vi "Startup Serial Packet Read.vi"(0 "VISA resource In":refnum<visa-resource-name>, 7 "End Character":string, 11 "error in":errorcluster) -> (4 "VISA resource Out":refnum<visa-resource-name>, 8 "Data Out":string, 15 "error out":errorcluster)   [LabVIEW 2014]
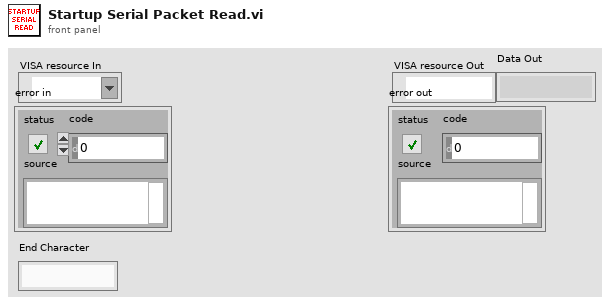
[diagram p1: front panel]
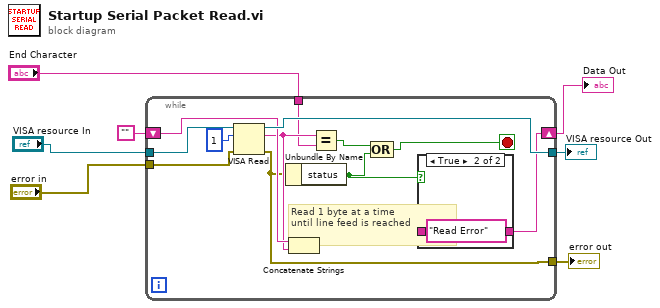
[diagram p0: block diagram]
diagram:
  n1 = while {
    tunnel: [w20] -> w3
    tunnel: [w14] -> w2
    tunnel: "VISA resource In" -> [w19]
    tunnel: "error in" -> [w18]
    shift-right: [w12] -> w6
    shift-left: "" -> [w17]
    tunnel: "End Character" -> [w8]
    stop <- w9 stop-if-true
    # "Read 1 byte at a time \nuntil line feed is reached"
    n2 = VISA Read(VISA resource name=w19, byte count=u32 1, error in (no error)=w18) -> (VISA resource name out=w20:refnum<visa-resource-name>, read buffer=w16:string, error out=w14:errorcluster)  [unwired: 1 out]
    n3 = Unbundle By Name(w14) -> ("status"=w11:bool)
    n4 = Concatenate Strings(w17, w16) -> (w13:string)
    n5 = Equal?(x=w16, y=w8) -> (x = y?=w10:bool)
    n6 = Compound Arithmetic op=OR(w10, w11) -> (w9:bool)
    n7 = case shown="True" w11 {
      tunnel: w13 -> [w21 _]
      tunnel: [w21 "Read Error"] -> w12
      frame False {
      }
      frame True {
      }
    }
  }
  "VISA resource Out" <- w3
  "error out" <- w2
  "Data Out" <- w6
